vi "LCM_read.vi"(8 "error in":errorcluster, 11 "LCM":T1={"connection ID"=refnum, "net address"=0, "port"=7667}) -> (0 "error out 2":errorcluster, 1 "data":string, 2 "ID":string, 3 "num":u32)   [LabVIEW 2015]
panel:
  out "Boolean":bool
  out "size":u32
  out "chanel":string
  out "seqnum":u32
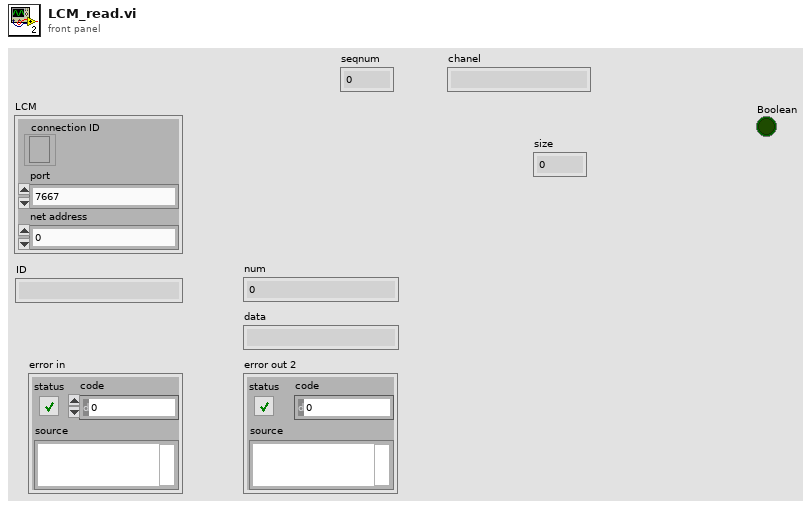
[diagram p1: front panel]
types:
  T1 = cluster{"connection ID":refnum<k16>, "net address":u32, "port":u16}
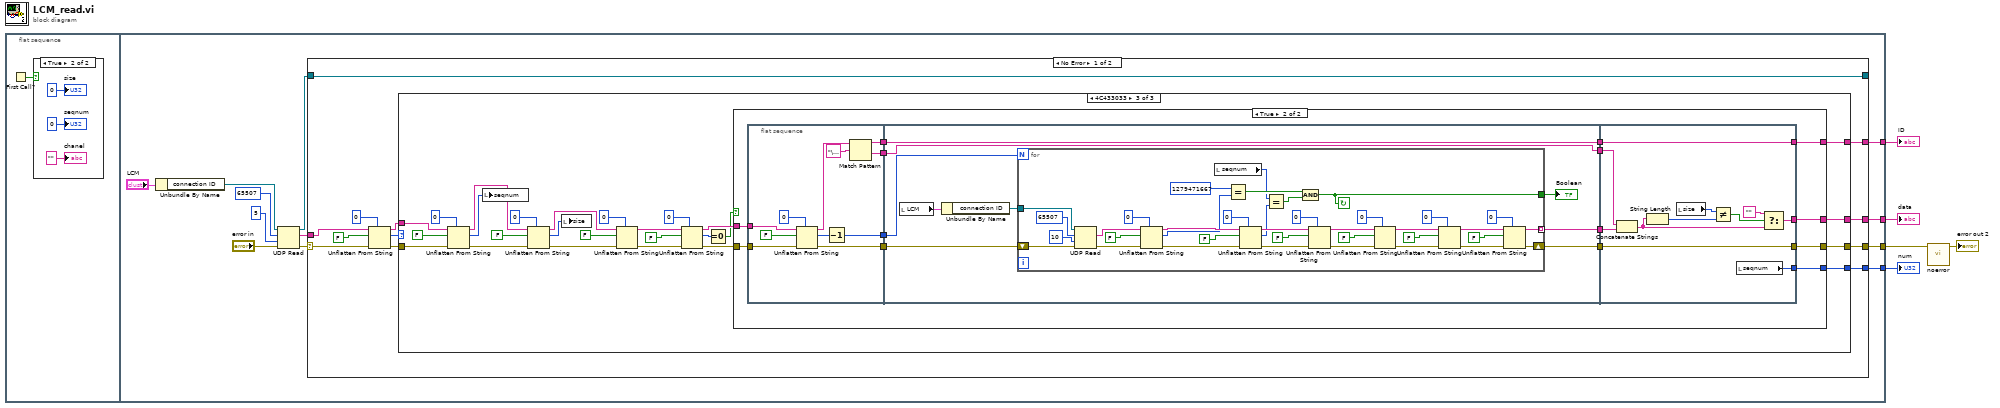
[diagram p0: block diagram]
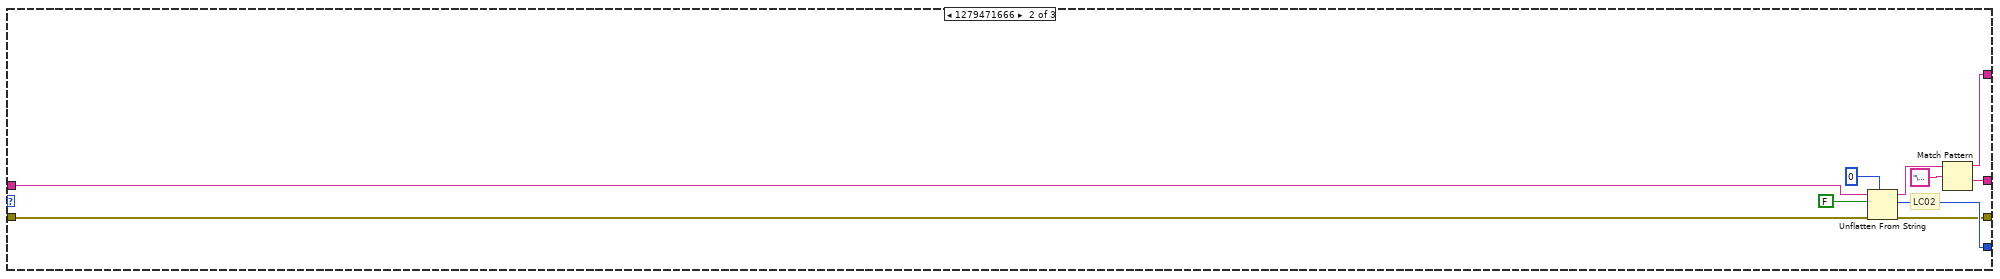
[diagram p4: hidden frame]
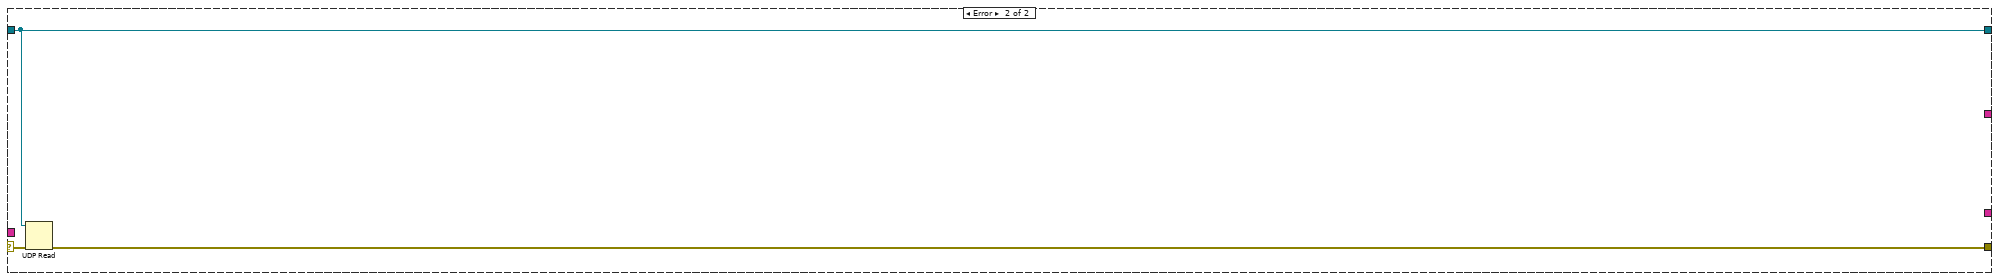
[diagram p6: hidden frame]
diagram:
  n1 = flat-sequence {
    tunnel: [w14] -> w5
    tunnel: [w13] -> w4
    tunnel: [w12] -> w2
    tunnel: [w11] -> w1
    frame #0 {
      n2 = First Call?() -> (First Call?: T/F=w6:bool)
      n3 = case shown="True" w6 {
        frame False {
        }
        frame True {
          "seqnum" <- u32 0
          "chanel" <- ""
          "size" <- u32 0 ("size")
        }
      }
    }
    frame #1 {
      n4 = Unbundle By Name("LCM") -> ("connection ID"=w10:refnum<k16>)
      n5 = UDP Read(connection ID=w10, max size (548)=65507, timeout ms (25000)=5, 8:"error in") -> (data out=w17:string, error out=w16:errorcluster, 3:w15:refnum<k16>)  [unwired: 2 out]
      n6 = case shown="No Error" w16 {
        selector: w16 -> [w29 w156]
        tunnel: w17 -> [w31 _]
        tunnel: [w25 w155] -> w13
        tunnel: [w22 w154] -> _
        tunnel: w15 -> [w22 w154]
        tunnel: [w28 _] -> w14
        tunnel: [w27 _] -> w12
        tunnel: [w26 _] -> w11
        frame No Error {
          n7 = Unflatten From String(type=u32 0, binary string=w31, data includes array or string size? (T)=FALSE, error in (no error)=w29) -> (rest of the binary string=w24:string, value=w30:u32, error out=w23:errorcluster)  [unwired: 1 in]
          n8 = case shown="4C433033" w30 {
            tunnel: [_ w40 w70] -> w28
            tunnel: [_ w41 w63] -> w27
            tunnel: [_ w38 w69] -> w26
            tunnel: [w34 w37 w68] -> w25
            tunnel: w24 -> [_ w36 w61]
            tunnel: w23 -> [w34 w35 w60]
            frame 0, Default {
            }
            frame 1279471666 {
              # "LC02"
              n9 = Unflatten From String(type=u32 0, binary string=w36, data includes array or string size? (T)=FALSE, error in (no error)=w35) -> (rest of the binary string=w44:string, value=w41:u32, error out=w37:errorcluster)  [unwired: 1 in]
              n10 = Match Pattern(string=w44, regular expression="\u0000") -> (before substring=w38:string, after substring=w40:string)  [unwired: 1 in, 2 out]
            }
            frame 1279471667 {
              n11 = Unflatten From String(type=u32 0, binary string=w61, data includes array or string size? (T)=FALSE, error in (no error)=w60) -> (rest of the binary string=w67:string, value=w62:u32, error out=w64:errorcluster)  [unwired: 1 in]
              n12 = local write "seqnum"(w62) -> ()
              n13 = Unflatten From String(type=u32 0, binary string=w67, data includes array or string size? (T)=FALSE, error in (no error)=w64) -> (rest of the binary string=w58:string, value=w45:u32, error out=w50:errorcluster)  [unwired: 1 in]
              n14 = local write "size"(w45) -> ()
              n15 = Unflatten From String(type=u32 0, binary string=w58, data includes array or string size? (T)=FALSE, error in (no error)=w50) -> (rest of the binary string=w54:string, error out=w49:errorcluster)  [unwired: 1 in, 1 out]
              n16 = Unflatten From String(type=u16 0, binary string=w54, data includes array or string size? (T)=FALSE, error in (no error)=w49) -> (rest of the binary string=w51:string, value=w47:u16, error out=w48:errorcluster)  [unwired: 1 in]
              n17 = Equal To 0?(x=w47) -> (x = 0?=w46:bool)
              n18 = case shown="True" w46 {
                tunnel: w51 -> [_ w85]
                tunnel: w48 -> [w71 w84]
                tunnel: [_ w80] -> w70
                tunnel: [w71 w79] -> w68
                tunnel: [_ w78] -> w69
                tunnel: [_ w77] -> w63
                frame False {
                }
                frame True {
                  n19 = flat-sequence {
                    tunnel: w85 -> [w96]
                    tunnel: w84 -> [w91]
                    tunnel: [w87] -> w83
                    tunnel: [w90] -> w82
                    tunnel: [w89] -> w75
                    tunnel: [w86] -> w73
                    tunnel: w83 -> [w105]
                    tunnel: w82 -> [w104]
                    tunnel: [w103] -> w81
                    tunnel: [w99] -> w76
                    tunnel: w75 -> [w99]
                    tunnel: [w98] -> w74
                    tunnel: w73 -> [w97]
                    tunnel: [w97] -> w72
                    tunnel: w81 -> [w152]
                    tunnel: [w153] -> w80
                    tunnel: [w152] -> w79
                    tunnel: [w145] -> w78
                    tunnel: [w146] -> w77
                    tunnel: w76 -> [w145]
                    tunnel: w74 -> [w144]
                    tunnel: w72 -> [w143]
                    frame #0 {
                      n20 = Unflatten From String(type=u16 0, binary string=w96, data includes array or string size? (T)=FALSE, error in (no error)=w91) -> (rest of the binary string=w92:string, value=w88:u16, error out=w90:errorcluster)  [unwired: 1 in]
                      n21 = Decrement(x=w88) -> (x-1=w87:u16)
                      n22 = Match Pattern(string=w92, regular expression="\u0000") -> (before substring=w89:string, after substring=w86:string)  [unwired: 1 in, 2 out]
                    }
                    frame #1 {
                      n23 = local read "LCM"() -> (w102:T1)
                      n24 = Unbundle By Name(w102) -> ("connection ID"=w101:refnum<k16>)
                      n25 = for {
                        N: w105 -> [_]
                        tunnel: w101 -> [w140]
                        shift-right: [w113] -> w103
                        shift-left: w104 -> [w139]
                        tunnel: [w112] -> w100
                        tunnel: [w106] -> w98 mode=indexing
                        stop <- w112 continue-if-true
                        n26 = UDP Read(connection ID=w140, max size (548)=65507, timeout ms (25000)=10, 8:w139) -> (data out=w107:string, error out=w118:errorcluster)  [unwired: 3 out]
                        n27 = Unflatten From String(type=u32 0, binary string=w107, data includes array or string size? (T)=FALSE, error in (no error)=w118) -> (rest of the binary string=w120:string, value=w114:u32, error out=w117:errorcluster)  [unwired: 1 in]
                        n28 = local read "seqnum"() -> (w108:u32)
                        n29 = Equal?(x=u32 1279471667, y=w114) -> (x = y?=w111:bool)
                        n30 = Unflatten From String(type=u32 0, binary string=w120, data includes array or string size? (T)=FALSE, error in (no error)=w117) -> (rest of the binary string=w119:string, value=w109:u32, error out=w116:errorcluster)  [unwired: 1 in]
                        n31 = Equal?(x=w108, y=w109) -> (x = y?=w110:bool)
                        n32 = Compound Arithmetic op=AND(w111, w110) -> (w112:bool)
                        n33 = Unflatten From String(type=u32 0, binary string=w119, data includes array or string size? (T)=FALSE, error in (no error)=w116) -> (rest of the binary string=w126:string, error out=w136:errorcluster)  [unwired: 1 in, 1 out]
                        n34 = Unflatten From String(type=u32 0, binary string=w126, data includes array or string size? (T)=FALSE, error in (no error)=w136) -> (rest of the binary string=w130:string, error out=w137:errorcluster)  [unwired: 1 in, 1 out]
                        n35 = Unflatten From String(type=u16 0, binary string=w130, data includes array or string size? (T)=FALSE, error in (no error)=w137) -> (rest of the binary string=w133:string, error out=w138:errorcluster)  [unwired: 1 in, 1 out]
                        n36 = Unflatten From String(type=u16 0, binary string=w133, data includes array or string size? (T)=FALSE, error in (no error)=w138) -> (rest of the binary string=w106:string, error out=w113:errorcluster)  [unwired: 1 in, 1 out]
                      }
                      "Boolean" <- w100
                    }
                    frame #2 {
                      n37 = Concatenate Strings(w143, w144) -> (w147:string)
                      n38 = String Length(string=w147) -> (length=w151:i32)
                      n39 = local read "size"() -> (w148:u32)
                      n40 = Not Equal?(x=w148, y=w151) -> (x != y?=w150:bool)
                      n41 = local read "seqnum"() -> (w146:u32)
                      n42 = Select(t="", s=w150, f=w147) -> (s? t:f=w153:string)
                    }
                  }
                }
              }
            }
          }
        }
        frame Error {
          n43 = UDP Read(connection ID=w154, 8:w156) -> (error out=w155:errorcluster)  [unwired: 1 in, 5 out]
        }
      }
    }
  }
  n44 = call "noerror.vi"("error in"=w4) -> ("error out"=→"error out 2":errorcluster)  [unwired: 10 in]
  "data" <- w5
  "num" <- w2
  "ID" <- w1
